vi "ResetSyncCards.vi"(0 "Array":refnum<k15>[](array[refnum])) -> ()   [LabVIEW 2014]
doc: "Resets Sync Cards. This is necessary when two seperate codes use the NI-sync cards."
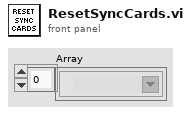
[diagram p1: front panel]
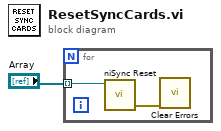
[diagram p0: block diagram]
diagram:
  n1 = for {
    tunnel: "Array" -> [w3] mode=indexing
    n2 = call <instrlib>:"niSync Reset.vi"("instrument handle"=w3) -> ("error out"=w2:errorcluster)  [unwired: 9 in, 1 out]
    n3 = call <vilib>:"Clear Errors.vi"("error in (no error)"=w2) -> ()  [unwired: 1 in, 6 out]
  }
